vi "Log BoP.vi"(9 "Stop Chat":bool, 10 "Send":bool, 11 "Enter Text":string) -> (3 "Chat Window":string)   [LabVIEW 2017]
uses:
  <vilib>/OPCUA/controls/Write Status.ctl
  <vilib>/OPCUA/controls/NodeId.ctl
  <vilib>/OPCUA/client/Multiple Write String.vi
  <vilib>/OPCUA/NI OPC UA Client.lvlib
panel:
  out "Log Loop":i32
  out "Send Loop":i32
  in  "Node Status":T1 items=["Good"=0, "Uncertain_InitialValue"=1083310080, "Uncertain_LastUsableValue"=1083179008, "Uncertain_SensorNotAccurate"=1083375616, "Uncertain_EngineeringUnitsExceeded"=1083441152, "Bad_NoCommunication"=2150694912, "Bad_NotReadable"=2151284736, "Bad_NotWritable"=2151350272, "Bad_OutOfRange"=2151415808, "Bad_WaitingForInitialData"=2150760448]
  in  "Time Stamp":timestamp
  in  "Node Status":T1 items=["Good"=0, "Uncertain_InitialValue"=1083310080, "Uncertain_LastUsableValue"=1083179008, "Uncertain_SensorNotAccurate"=1083375616, "Uncertain_EngineeringUnitsExceeded"=1083441152, "Bad_NoCommunication"=2150694912, "Bad_NotReadable"=2151284736, "Bad_NotWritable"=2151350272, "Bad_OutOfRange"=2151415808, "Bad_WaitingForInitialData"=2150760448]
  in  "Time Stamp":timestamp
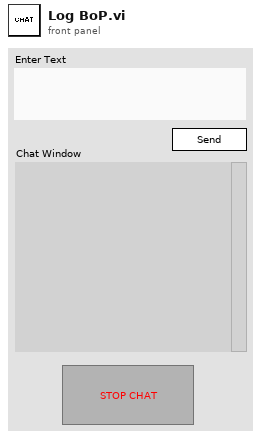
[diagram p1: front panel]
types:
  T1 = typedef "Write Status.ctl" = u32
  T2 = enum16{"open", "replace", "create", "open or create", "replace or create", "replace or create with confirmation"}
  T3 = typedef "OPC UA Client Refnum.ctl" = refnum<k21>
  T4 = typedef "NodeId.ctl" = string
  T5 = cluster{"node ID":T4, "value":string, "timestamp (current time)":timestamp, "node status":T1}
  T6 = cluster{"node ID":T4, "value":string, "timestamp (current time)":timestamp, "node status":T1}[]
  T7 = typedef "Subscription ID.ctl" = u32
  T8 = typedef "Subscription Data Change.ctl" = cluster{"node ID":T4, " value":variant, "timestamp":timestamp, "data type":T9, "status code":T10}
  T9 = typedef "Data Type.ctl" = u16
  T10 = typedef "OPC UA StatusCode.ctl" = u32
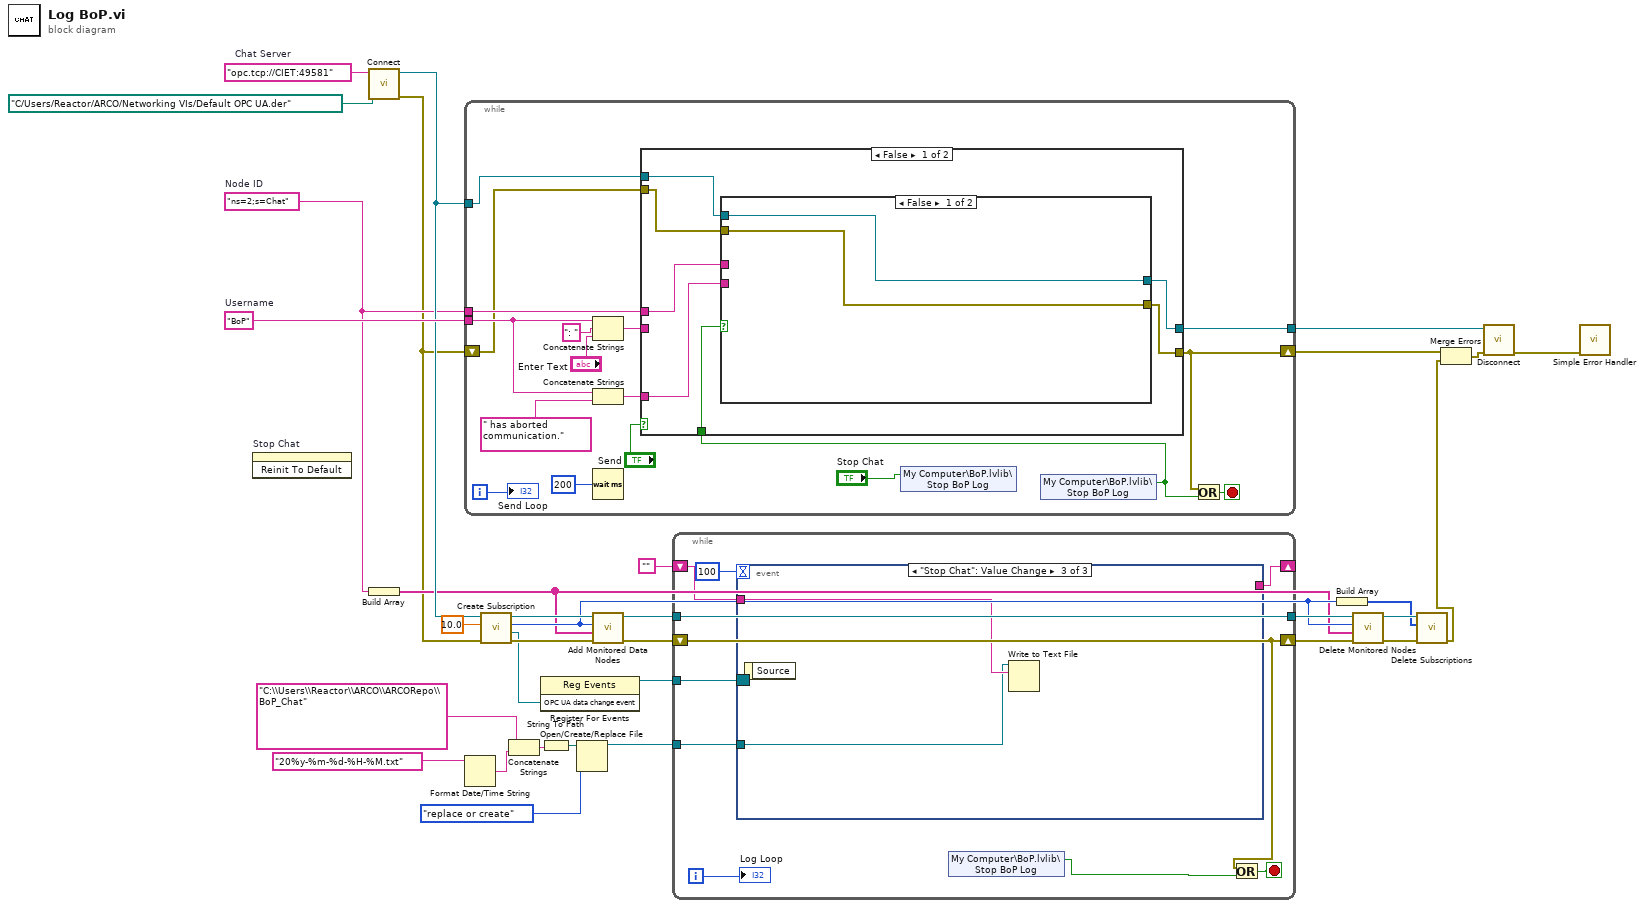
[diagram p0: block diagram]
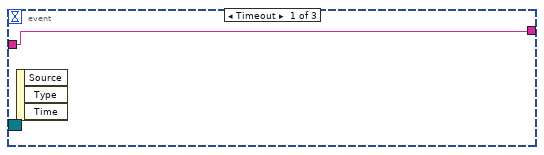
[diagram p2: hidden frame]
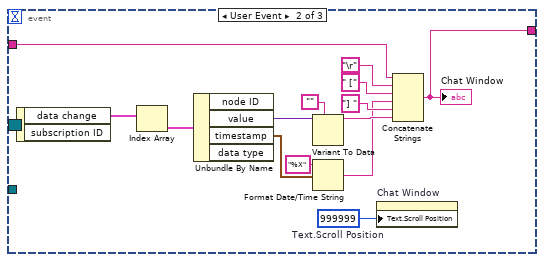
[diagram p3: hidden frame]
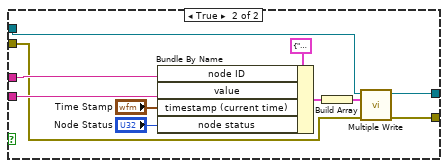
[diagram p4: hidden frame]
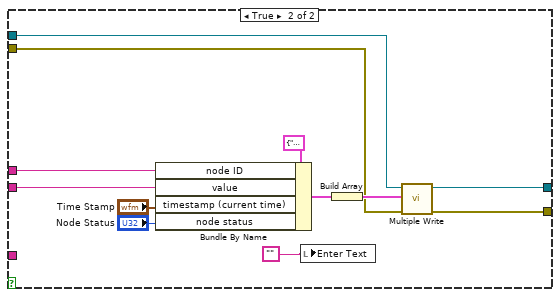
[diagram p5: hidden frame]
diagram:
  w16 = "ns=2;s=Chat"  # Node ID
  w31 = "BoP"  # Username
  w32 = "opc.tcp://CIET:49581"  # Chat Server
  n1 = invoke on="Stop Chat" class="Bool (strict)" method="Reinit To Default"() -> ()  [unwired: 3 in, 3 out]
  n2 = call <vilib>:"Connect.vi"("client certificate file"=path "C:/Users/Reactor/ARCO/Networking VIs/Default OPC UA.der", "server endpoint URL"=w32) -> ("error out"=w6:errorcluster, "OPC UA client refnum out"=w30:T3)  [unwired: 7 in, 1 out]
  n3 = Build Array(w16) -> (w15:string[])
  n4 = while {
    tunnel: w16 -> [w42]
    tunnel: w31 -> [w47]
    tunnel: w30 -> [w40]
    tunnel: [w41] -> w13
    shift-right: [w36] -> w1
    shift-left: w6 -> [w39]
    i -> [w45]
    stop <- w37 stop-if-true
    n5 = Concatenate Strings(w47, ": ", "Enter Text") -> (w43:string)
    n6 = Concatenate Strings(w47, " has aborted communication.") -> (w38:string)
    n7 = Wait (ms)(milliseconds to wait=u32 200) -> ()  [unwired: 1 out]
    n8 = shared-variable "My Computer\\BoP.lvlib\\Stop BoP Log"("Stop Chat") -> ()  [unwired: 1 in, 1 out]
    n9 = shared-variable "My Computer\\BoP.lvlib\\Stop BoP Log"() -> (w34:bool)  [unwired: 1 in, 1 out]
    n10 = case shown="False" "Send" {
      tunnel: w43 -> [_ w77]
      tunnel: w42 -> [w55 w76]
      tunnel: [w51 w74] -> w41
      tunnel: [w52 w73] -> w36
      tunnel: w40 -> [w53 w72]
      tunnel: w39 -> [w54 w71]
      tunnel: w34 -> [w57 _]
      tunnel: w38 -> [w56 _]
      frame False {
        n11 = case shown="False" w57 {
          tunnel: w56 -> [_ w65]
          tunnel: w55 -> [_ w64]
          tunnel: w54 -> [w58 w63]
          tunnel: w53 -> [w59 w62]
          tunnel: [w59 w61] -> w51
          tunnel: [w58 w60] -> w52
          frame False {
          }
          frame True {
            n12 = Bundle By Name(cluster=T5 {"node ID"="", "value"="", "timestamp (current time)"=timestamp(0 s since 1904-01-01), "node status"=0} ("request"), "node ID"=w64, "value"=w65, "timestamp (current time)"="Time Stamp", "node status"="Node Status") -> (w68:T5)
            n13 = Build Array(w68) -> (w67:T6)
            n14 = call-poly <vilib>:"Multiple Write.vi"("error in (no error)"=w63, "requests"=w67, "OPC UA client refnum in"=w62) -> ("error out"=w60:errorcluster, "OPC UA client refnum out"=w61:T3)  [unwired: 5 in, 2 out]
          }
        }
      }
      frame True {
        n15 = Bundle By Name(cluster=T5 {"node ID"="", "value"="", "timestamp (current time)"=timestamp(0 s since 1904-01-01), "node status"=0} ("request"), "node ID"=w76, "value"=w77, "timestamp (current time)"="Time Stamp", "node status"="Node Status") -> (w80:T5)
        n16 = local write "Enter Text"("") -> ()
        n17 = Build Array(w80) -> (w79:T6)
        n18 = call-poly <vilib>:"Multiple Write.vi"("error in (no error)"=w71, "requests"=w79, "OPC UA client refnum in"=w72) -> ("error out"=w73:errorcluster, "OPC UA client refnum out"=w74:T3)  [unwired: 5 in, 2 out]
      }
    }
    n19 = Or(x=w36, y=w34) -> (x .or. y?=w37:bool)
    "Send Loop" <- w45
  }
  n20 = Format Date/Time String(time format string (%c)="20%y-%m-%d-%H-%M.txt") -> (date/time string=w10:string)  [unwired: 2 in]
  n21 = call <vilib>:"Create Subscription.vi"("error in (no error)"=w6, "publishing interval (1000 ms)"=10.0, "OPC UA client refnum in"=w30) -> ("error out"=w28:errorcluster, "OPC UA data change event"=w27:refnum<user-event>, "subscription ID out"=w19:T7, "OPC UA client refnum out"=w29:T3)  [unwired: 4 in, 1 out]
  n22 = Concatenate Strings("C:\\Users\\Reactor\\ARCO\\ARCORepo\\BoP_Chat", w10) -> (w8:string)
  n23 = register-events(w27) -> (reference out=w26:refnum<event-registration>)  [unwired: 2 in, 1 out]
  n24 = String To Path(string=w8) -> (path=w7:path)
  n25 = Open/Create/Replace File(file path (use dialog)=w7, operation (0:open)=T2."replace or create") -> (refnum out=w17:refnum<file>)  [unwired: 4 in, 2 out]
  n26 = call <vilib>:"Add Monitored Data Nodes.vi"("error in (no error)"=w28, "node IDs"=w15, "subscription ID in"=w19, "OPC UA client refnum in"=w29) -> ("error out"=w22:errorcluster, "OPC UA client refnum out"=w24:T3)  [unwired: 4 in, 2 out]
  n27 = while {
    tunnel: w26 -> [w92]
    shift-right: [w90] -> _
    shift-left: "" -> [w91]
    tunnel: w24 -> [w89]
    tunnel: [w89] -> w23
    tunnel: w17 -> [w88]
    shift-right: [w84] -> w5
    shift-left: w22 -> [w84]
    i -> [w87]
    stop <- w85 stop-if-true
    n28 = event shown="[2] \"Stop Chat\": Value Change" {
      selector: w92 -> [_ _ _]
      dyn-events: _ -> [_ _ _]
      timeout: 100 -> [_ _ _]
      tunnel: w91 -> [w93 w96 w109]
      tunnel: [w93 w95 _] -> w90
      tunnel: w88 -> [_ _ w108]
      event Timeout {
        n29 = event-data() -> ()  [unwired: 1 in, 3 out]
      }
      event User Event {
        w94 = u32 999999  # Text.Scroll Position
        n30 = event-data() -> ("data change"=w107:T8[])  [unwired: 1 in, 1 out]
        n31 = Index Array(array=w107) -> (element=w106:T8)  [unwired: 1 in]
        n32 = Unbundle By Name(w106) -> ("value"=w105:variant, "timestamp"=w103:timestamp)  [unwired: 2 out]
        n33 = Variant To Data(type="", Variant=w105) -> (data=w101:string)  [unwired: 1 in, 1 out]
        n34 = Format Date/Time String(time format string (%c)="%X", seconds (now)=w103) -> (date/time string=w99:string)  [unwired: 1 in]
        n35 = property on="Chat Window" class="Str"("Text.Scroll Position"=w94) -> ()  [unwired: 2 in, 2 out]
        n36 = Concatenate Strings(w96, "\r", " [", w99, "] ", w101) -> (w95:string)
        "Chat Window" <- w95
      }
      event "Stop Chat": Value Change {
        n37 = event-data() -> ()  [unwired: 1 in, 1 out]
        n38 = Write to Text File(file (use dialog)=w108, text=w109) -> ()  [unwired: 2 in, 3 out]
      }
    }
    n39 = shared-variable "My Computer\\BoP.lvlib\\Stop BoP Log"() -> (w83:bool)  [unwired: 1 in, 1 out]
    n40 = Or(x=w84, y=w83) -> (x .or. y?=w85:bool)
    "Log Loop" <- w87
  }
  n41 = Build Array(w19) -> (w18:T7[])
  n42 = call <vilib>:"Delete Monitored Nodes.vi"("error in (no error)"=w5, "node IDs"=w15, "subscription ID in"=w19, "OPC UA client refnum in"=w23) -> ("error out"=w20:errorcluster, "OPC UA client refnum out"=w21:T3)  [unwired: 3 in, 3 out]
  n43 = call <vilib>:"Delete Subscriptions.vi"("error in (no error)"=w20, "subscription IDs"=w18, "OPC UA client refnum in"=w21) -> ("error out"=w2:errorcluster)  [unwired: 6 in, 2 out]
  n44 = Merge Errors(w1, w2) -> (w3:errorcluster)
  n45 = call <vilib>:"Disconnect.vi"("error in (no error)"=w3, "OPC UA client refnum in"=w13) -> ("error out"=w33:errorcluster)  [unwired: 9 in]
  n46 = call <vilib>:"Simple Error Handler.vi"("error in (no error)"=w33) -> ()  [unwired: 4 in, 5 out]
